vi "Button To Toggle Vr3.vi"(1 "InValue":bool) -> (0 "Result":bool)   [LabVIEW 2012]
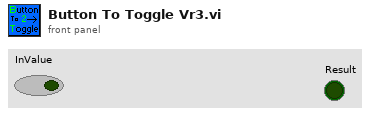
[diagram p1: front panel]
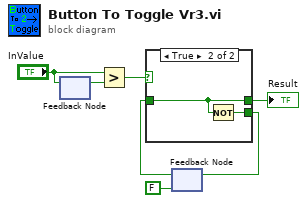
[diagram p0: block diagram]
diagram:
  n1 = feedback #1() -> (w7:bool)  [unwired: 1 in]
  n2 = feedback-in #1("InValue") -> ()
  n3 = Greater?(x="InValue", y=w7) -> (0:w5:bool)
  n4 = feedback #2(FALSE) -> (w3:bool)
  n5 = case shown="True" w5 {
    tunnel: w3 -> [w8 w9]
    tunnel: [w8 w10] -> w2
    tunnel: [w8 w9] -> w1
    frame False {
    }
    frame True {
      n6 = Not(x=w9) -> (.not. x?=w10:bool)
    }
  }
  "Result" <- w1
  n7 = feedback-in #2(w2) -> ()
